vi "setBasePath.vi"(8 "error in":errorcluster, 10 "base path":path, 11 "camera in":refnum<class "camera.lvclass">) -> (0 "error out":errorcluster)   [LabVIEW 2020, in "camera.lvclass"]
uses:
  camera.lvclass
  camera.lvclass/camera.ctl
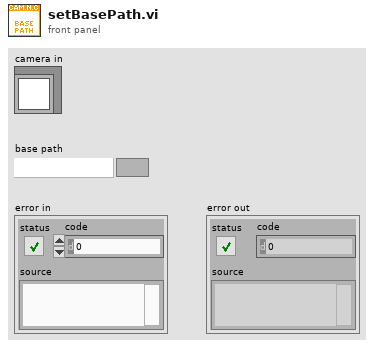
[diagram p1: front panel]
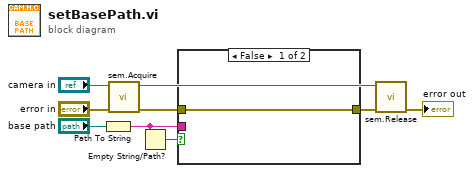
[diagram p0: block diagram]
diagram:
  n1 = Path To String(path="base path") -> (string=w1:string)
  n2 = call "sem.Acquire.vi"("error in"="error in", "camera.nit in"="camera in") -> ("error out"=w5:errorcluster)  [unwired: 9 in]
  n3 = Empty String/Path?(string/path=w1) -> (empty?=w3:bool)
  n4 = case shown="False" w3 {
    tunnel: w1 -> [_ _]
    tunnel: w5 -> [w9 w10]
    tunnel: [w9 w10] -> w4
    frame False {
    }
    frame True {
    }
  }
  n5 = call "sem.Release.vi"("error in"=w4, "camera.nit in"="camera in") -> ("error out"=→"error out":errorcluster)  [unwired: 9 in]
